vi "GetLidarDistance.vi"() -> ()   [LabVIEW 2017]
panel:
  in  "error in":errorcluster
  out "(hi.lo)":u16
  out "error out":errorcluster
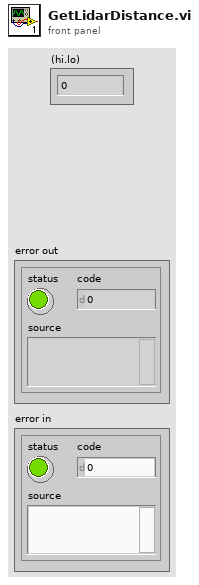
[diagram p1: front panel]
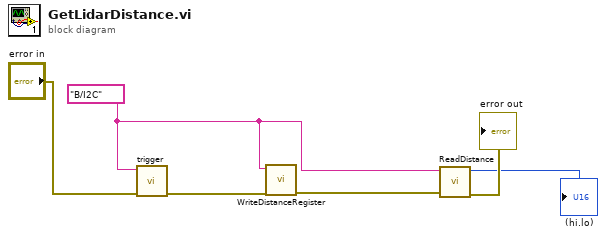
[diagram p0: block diagram]
diagram:
  w1 = tag "B/I2C" ("Channel Name")
  n1 = call "trigger.vi"("error in (no error)"="error in", "Channel Name"=w1) -> ("error out"=w6:errorcluster)  [unwired: 9 in]
  n2 = call "WriteDistanceRegister.vi"("error in (no error)"=w6, "Channel Name"=w1) -> ("error out"=w5:errorcluster)  [unwired: 9 in]
  n3 = call "ReadDistance.vi"("error in (no error)"=w5, "Channel Name"=w1) -> ("error out"=→"error out":errorcluster, "(hi.lo)"=→"(hi.lo)":u16)  [unwired: 8 in]
